vi "Read FC1 ILC Serial Settings.vi"(8 "error in (no error)":errorcluster, 11 "Boot Loader in":refnum<class "Boot Loader.lvclass">) -> (0 "error out":errorcluster, 2 "ILC Serial Settings":T1={"Serial"={"Serial Protocol"=enum."RS485", "Protocol Parameters"={"VISA resource name"="", "Baud Rate"=9600, "Data Bits"=8, "Parity"=enum."None", "Flow Control"=0, "Stop Bits"=10, "Timeout (ms)"=10000}, "Serial Message Parameters"={"Byte Count"=200, "Enable Termination Character"=FALSE, "Termination Char"=200}}} {"Serial"."Serial Message Parameters"."Termination Char" format="%x"; "Serial"."Protocol Parameters"."Stop Bits" items=["1.0"=10, "1.5"=15, "2.0"=20]; "Serial"."Protocol Parameters"."Flow Control" items=["None", "XON/XOFF", "RTS/CTS", "XON/XOFF & RTS/CTS", "DTR/DSR", "XON/XOFF & DTR/DSR"]; "Serial"."Protocol Parameters"."Data Bits" min=5 max=8 step=1}, 3 "Boot Loader out":refnum<class "Boot Loader.lvclass">)   [LabVIEW 2015, in "Boot Loader.lvclass"]
uses:
  Boot Loader.lvclass
  <userlib>/Common/ILC/Configuration/Serial.ctl
  <userlib>/Common/SerialProtocols/Configuration/SerialConfig.ctl
  <userlib>/Common/SerialProtocols/Configuration/SerialProtocol.ctl
  <userlib>/Common/SerialProtocols/Configuration/ProtocolParameters.ctl
  <userlib>/Common/SerialProtocols/Configuration/SerialMessageParameters.ctl
  Typedefs/Serial Settings.ctl
  Typedefs/Connection Settings.ctl
  Settings/Settings.lvclass
  Typedefs/FAMT Typedefs.lvlib
  <userlib>/Common/SerialProtocols/SerialProtocols.lvlib
  <userlib>/Common/ILC/Configuration/ILCConfiguration.lvlib
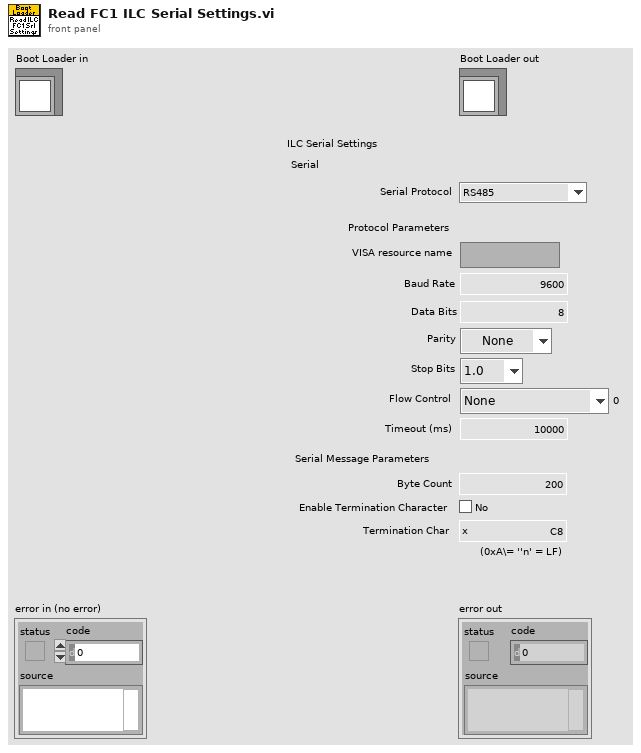
[diagram p1: front panel]
types:
  T1 = typedef "ILCCommon.lvlib/ILCConfiguration.lvlib/Serial.ctl" = cluster{"Serial":T2}
  T2 = typedef "SerialProtocols.lvlib/SerialConfig.ctl" = cluster{"Serial Protocol":T3, "Protocol Parameters":T4, "Serial Message Parameters":T5}
  T3 = typedef "SerialProtocols.lvlib/SerialProtocol.ctl" = enum16{"RS232", "RS485", "SerialSimulator"}
  T4 = typedef "SerialProtocols.lvlib/ProtocolParameters.ctl" = cluster{"VISA resource name":refnum<visa-resource-name>, "Baud Rate":u32, "Data Bits":u16, "Parity":enum16{"None", "Odd", "Even", "Mark", "Space"}, "Flow Control":u16, "Stop Bits":u16, "Timeout (ms)":u32}
  T5 = typedef "SerialProtocols.lvlib/SerialMessageParameters.ctl" = cluster{"Byte Count":u32, "Enable Termination Character":bool, "Termination Char":u8}
  T6 = typedef "FAMT Typedefs.lvlib/Connection Settings.ctl" = cluster{"Pressure Servo Valve 1 DAC":u8, "Pressure Servo Valve 2 DAC":u8, "Flow Control Valve DAC":u8, "Load Cell ADC":u8, "FC1 ILC Port":refnum<visa-resource-name>, "FC2 ILC Port":refnum<visa-resource-name>, "Tovey A-B Port":refnum<visa-resource-name>, "Tovey C-D Port":refnum<visa-resource-name>, "Tovey E-F Port":refnum<visa-resource-name>, "FC1 ILC Protocol":T3, "FC2 ILC Protocol":T3, "Tovey A-B Protocol":T3, "Tovey C-D Protocol":T3, "Tovey E-F Protocol":T3}
  T7 = typedef "FAMT Typedefs.lvlib/Serial Settings.ctl" = cluster{"Baud Rate":u32, "Data Bits":u16, "Parity":enum16{"None", "Odd", "Even", "Mark", "Space"}, "Flow Control":u16, "Stop Bits":u16, "Timeout (ms)":u32, "Byte Count":u32, "Enable Termination Character":bool, "Termination Char":u8}
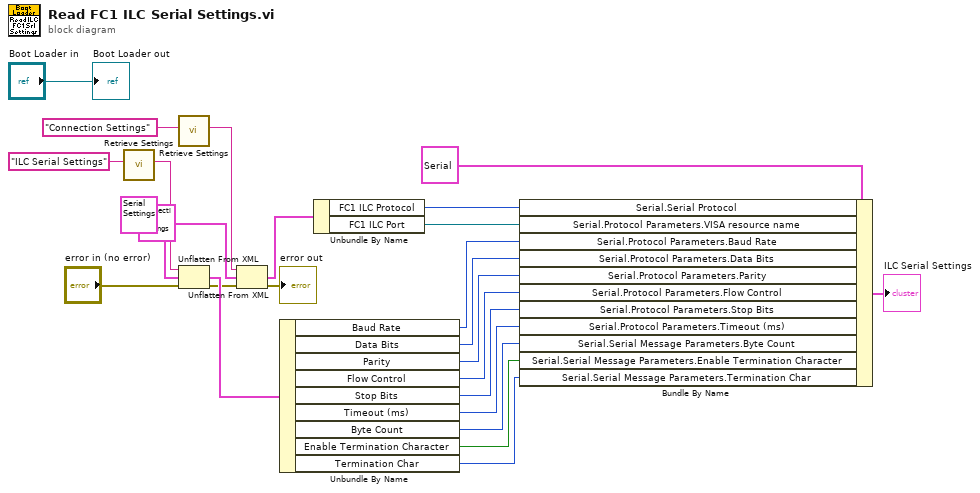
[diagram p0: block diagram]
diagram:
  n1 = call "Retrieve Settings.vi"("configName"="ILC Serial Settings") -> ("xmlConfig"=w24:string)  [unwired: 8 in, 2 out]
  n2 = call "Retrieve Settings.vi"("configName"="Connection Settings") -> ("xmlConfig"=w9:string)  [unwired: 8 in, 2 out]
  n3 = Unflatten From XML(xml string=w24, type=T7 {"Baud Rate"=9600, "Data Bits"=8, "Parity"=enum."None", "Flow Control"=0, "Stop Bits"=10, "Timeout (ms)"=10000, "Byte Count"=200, "Enable Termination Character"=FALSE, "Termination Char"=200} ("Serial Settings"), error in (no error)="error in (no error)") -> (value=w20:T7, error out=w3:errorcluster)
  n4 = Unflatten From XML(xml string=w9, type=T6 {"Pressure Servo Valve 1 DAC"=1, "Pressure Servo Valve 2 DAC"=2, "Flow Control Valve DAC"=3, "Load Cell ADC"=1, "FC1 ILC Port"="", "FC2 ILC Port"="", "Tovey A-B Port"="", "Tovey C-D Port"="", "Tovey E-F Port"="", "FC1 ILC Protocol"=enum."SerialSimulator", "FC2 ILC Protocol"=enum."SerialSimulator", "Tovey A-B Protocol"=enum."SerialSimulator", "Tovey C-D Protocol"=enum."SerialSimulator", "Tovey E-F Protocol"=enum."SerialSimulator"} ("Connection Settings"), error in (no error)=w3) -> (value=w7:T6, error out=→"error out":errorcluster)
  n5 = Unbundle By Name(w20) -> ("Baud Rate"=w11:u32, "Data Bits"=w12:u16, "Parity"=w13:enum16{"None", "Odd", "Even", "Mark", "Space"}, "Flow Control"=w14:u16, "Stop Bits"=w15:u16, "Timeout (ms)"=w16:u32, "Byte Count"=w17:u32, "Enable Termination Character"=w18:bool, "Termination Char"=w19:u8)
  n6 = Unbundle By Name(w7) -> ("FC1 ILC Protocol"=w6:T3, "FC1 ILC Port"=w5:refnum<visa-resource-name>)
  n7 = Bundle By Name(cluster=T1 {"Serial"={"Serial Protocol"=enum."RS232", "Protocol Parameters"={"VISA resource name"="", "Baud Rate"=0, "Data Bits"=0, "Parity"=enum."None", "Flow Control"=0, "Stop Bits"=0, "Timeout (ms)"=0}, "Serial Message Parameters"={"Byte Count"=0, "Enable Termination Character"=FALSE, "Termination Char"=0}}} ("ILC"), "Serial.Serial Protocol"=w6, "Serial.Protocol Parameters.VISA resource name"=w5, "Serial.Protocol Parameters.Baud Rate"=w11, "Serial.Protocol Parameters.Data Bits"=w12, "Serial.Protocol Parameters.Parity"=w13, "Serial.Protocol Parameters.Flow Control"=w14, "Serial.Protocol Parameters.Stop Bits"=w15, "Serial.Protocol Parameters.Timeout (ms)"=w16, "Serial.Serial Message Parameters.Byte Count"=w17, "Serial.Serial Message Parameters.Enable Termination Character"=w18, "Serial.Serial Message Parameters.Termination Char"=w19) -> (→"ILC Serial Settings":T1)
  "Boot Loader out" <- "Boot Loader in"
